vi "Large Time Scale Integration Check.vi"() -> ()   [LabVIEW 2009]
panel:
  out "18b (s-fxp-1) out":fxp<+/-,18,1> format="%.18g"
  in  "Integrand":fxp<+/-,18,1> format="%.18g"
  in  "Size of Integrator":fxp<+,6,6>
  in  "stop":bool
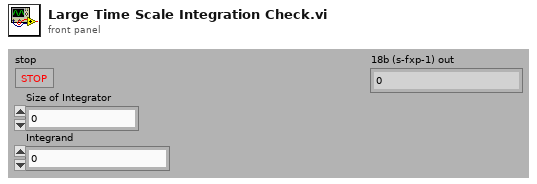
[diagram p1: front panel]
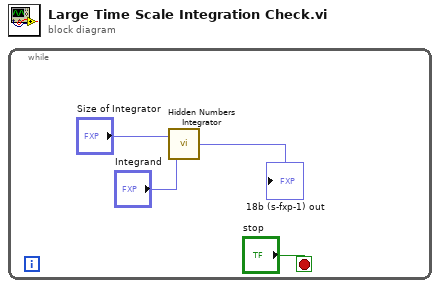
[diagram p0: block diagram]
diagram:
  n1 = while {
    stop <- "stop" stop-if-true
    n2 = call "Hidden Numbers Integrator.vi"("Integrand"="Integrand", "Size of Integrator"="Size of Integrator") -> ("18b (s-fxp-1) out"=→"18b (s-fxp-1) out":fxp<+/-,18,1>)
  }
